vi "MainLogging.vi"() -> ()   [LabVIEW 2020]
uses:
  510ae374-dab3-4fa4-a969-3b7666ba4ceb.vi
  5b4dafd0-0cd6-4d81-9f73-653c943f8121.vi
  <vilib>/Array/Sort 2D Array - Pop Stack.vi
  <vilib>/Array/Sort 2D Array - Push Stack.vi
  510ae374-dab3-4fa4-a969-3b7666ba4ceb.vi/269d4b3b-47f5-49e3-8884-44851e4dd9d5.vi
  510ae374-dab3-4fa4-a969-3b7666ba4ceb.vi/6d99389c-673d-4efb-bf33-19b32bcf4cf8.vi
  5b4dafd0-0cd6-4d81-9f73-653c943f8121.vi/269d4b3b-47f5-49e3-8884-44851e4dd9d5.vi
  5b4dafd0-0cd6-4d81-9f73-653c943f8121.vi/6d99389c-673d-4efb-bf33-19b32bcf4cf8.vi
  Global Variables/Global Enable Logging.vi
panel:
  out "Logging":bool
  out "Display Duration":dbl[](array[numeric])
  out "Square Timestamp":dbl[](array[numeric])
  out "Square Position":dbl[](array[numeric])
  out "Square Size":dbl[](array[numeric])
  out "Avg Pupil Size Right Before NN":dbl[](array[numeric])
  out "Avg Pupil Size Left Before NN":dbl[](array[numeric])
  out "Answer":dbl[](array[numeric])
  out "Label":dbl[](array[numeric])
  out "Classification":dbl[](array[numeric])
  out "Frame Rate":dbl[](array[numeric])
  out "Window Size":dbl[](array[numeric])
  out "Right Pupil Window Avg":dbl[](array[numeric])
  out "Left Pupil Window Avg":dbl[](array[numeric])
  out "Window TimeStamp":dbl[](array[numeric])
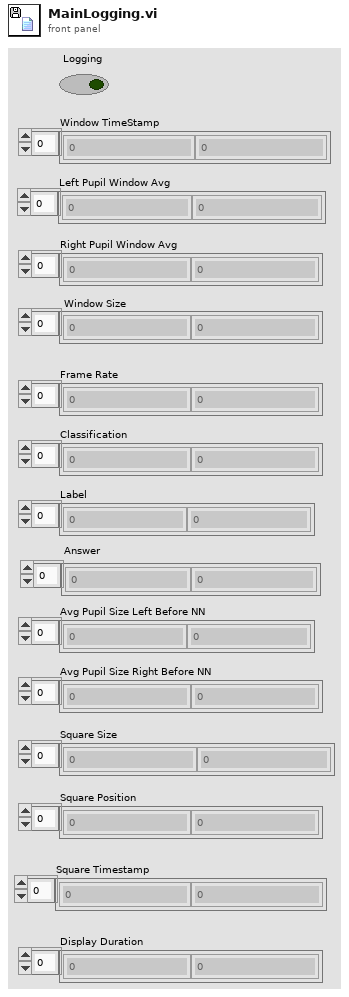
[diagram p1: front panel]
types:
  T1 = enum16{"open", "replace", "create", "open or create", "replace or create", "replace or create with confirmation"}
  T2 = cluster{"[0]":refnum<file>, "[1]":refnum<file>, "[2]":refnum<file>, "[3]":refnum<file>, "[4]":refnum<file>, "[5]":refnum<file>, "[6]":refnum<file>, "[7]":refnum<file>, "[8]":refnum<file>, "[9]":refnum<file>, "[10]":refnum<file>, "[11]":refnum<file>, "[12]":refnum<file>, "[13]":refnum<file>, "[14]":refnum<file>}
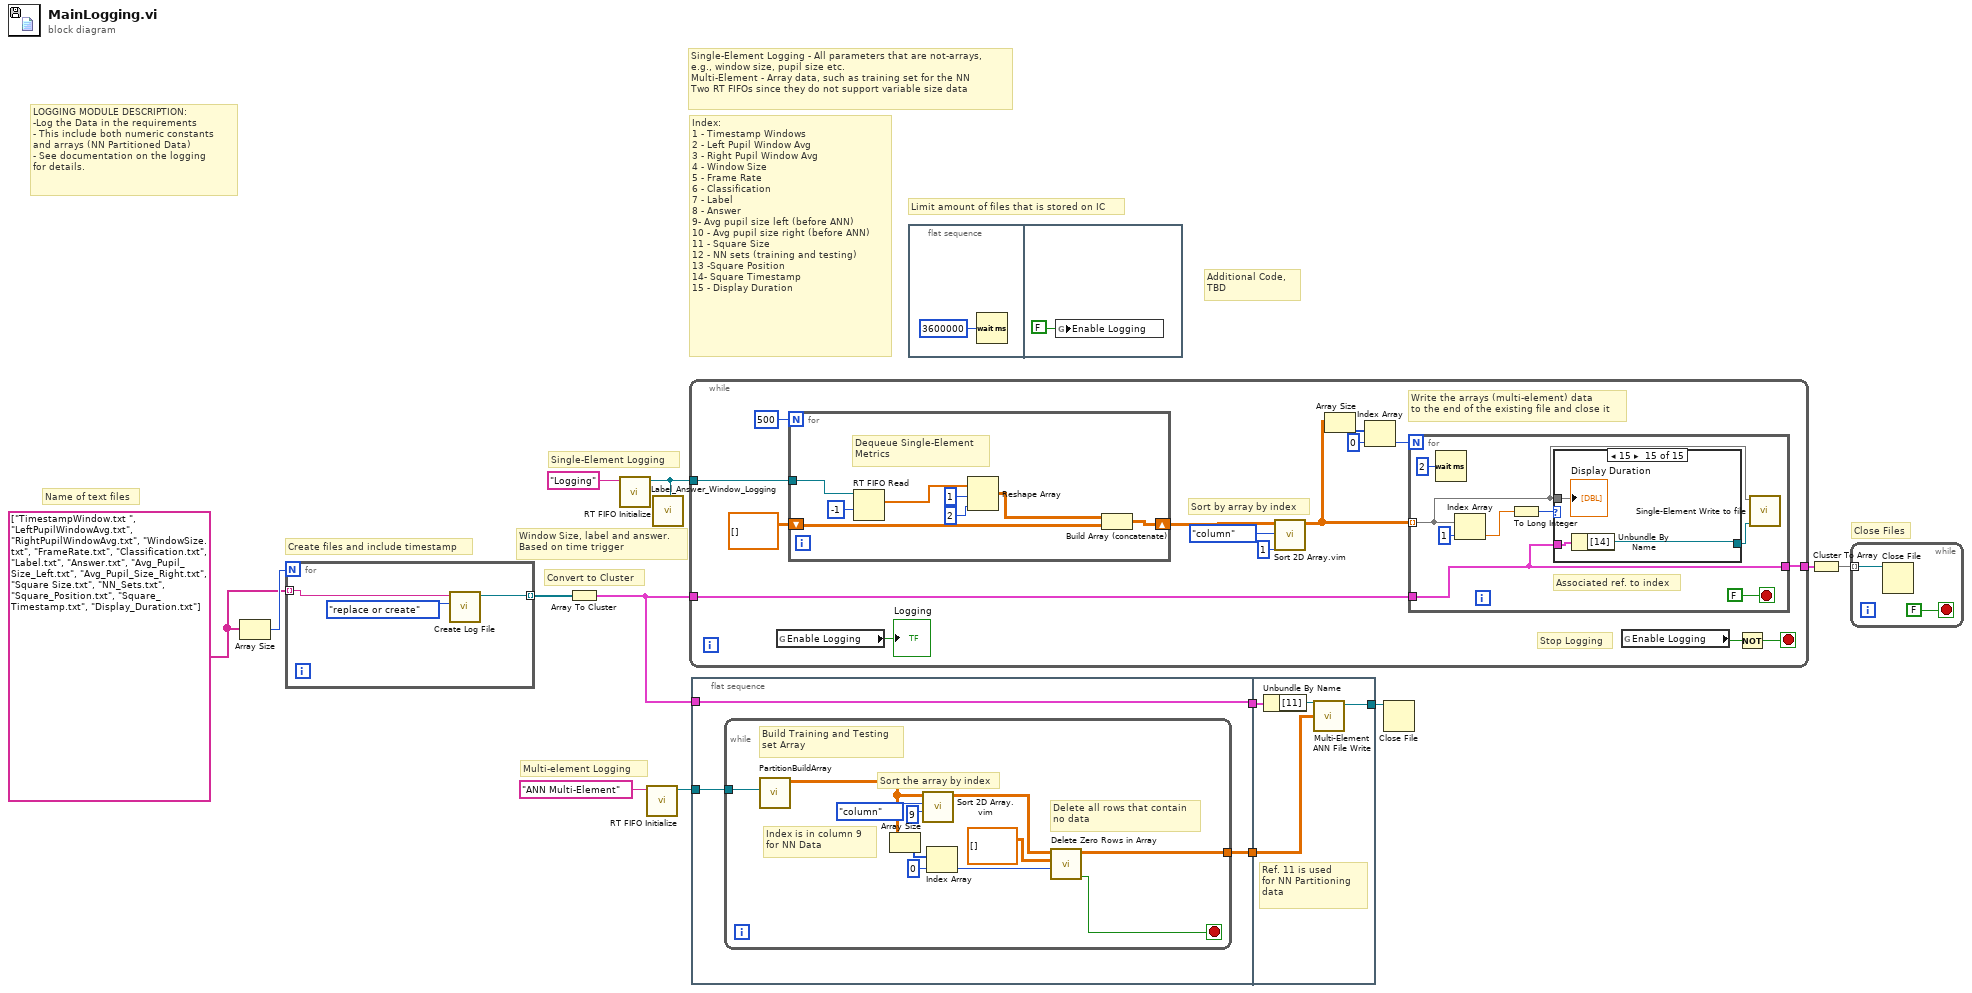
[diagram p0: block diagram]
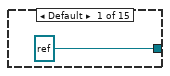
[diagram p2: hidden frame]
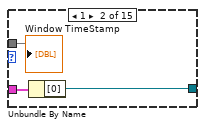
[diagram p3: hidden frame]
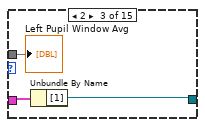
[diagram p4: hidden frame]
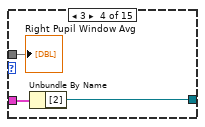
[diagram p5: hidden frame]
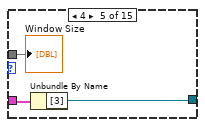
[diagram p6: hidden frame]
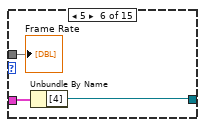
[diagram p7: hidden frame]
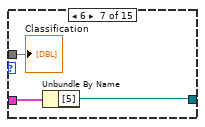
[diagram p8: hidden frame]
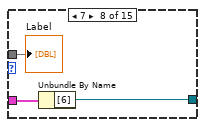
[diagram p9: hidden frame]
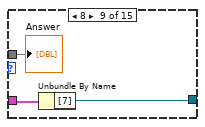
[diagram p10: hidden frame]
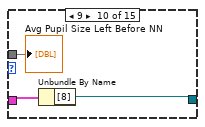
[diagram p11: hidden frame]
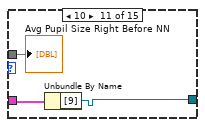
[diagram p12: hidden frame]
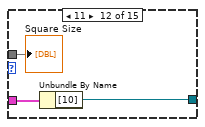
[diagram p13: hidden frame]
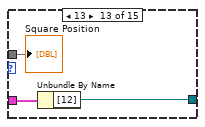
[diagram p14: hidden frame]
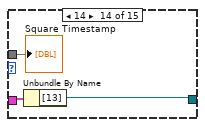
[diagram p15: hidden frame]
diagram:
  w8 = string[] ["TimestampWindow.txt ", "LeftPupilWindowAvg.txt", "RightPupilWindowAvg.txt", "WindowSize.txt", "FrameRate.txt", "Classification.txt", "Label.txt", "Answer.txt", "Avg_Pupil_Size_Left.txt", "Avg_Pupil_Size_Right.txt", "Square Size.txt", "NN_Sets.txt", "Square_Position.txt", "Square_Timestamp.txt", "Display_Duration.txt"]
  # "Close Files"
  # "LOGGING MODULE DESCRIPTION: \n-Log the Data in the requirements \n- This include both numeric constants \nand arrays (NN Partitioned Data) \n- See documentation on the logging \nfor details."
  # "Convert to Cluster"
  # "Additional Code, \nTBD"
  # "Name of text files"
  # "Multi-element Logging"
  # "Create files and include timestamp"
  # "Limit amount of files that is stored on IC"
  # "Window Size, label and answer. \nBased on time trigger"
  # "Single-Element Logging - All parameters that are not-arrays, \ne.g., window size, pupil size etc. \nMulti-Element - Array data, such as training set for the NN \nTwo RT FIFOs since they do not support variable size data"
  # "Single-Element Logging"
  # "Index: \n1 - Timestamp Windows \n2 - Left Pupil Window Avg \n3 - Right Pupil Window Avg\n4 - Window Size\n5 - Frame Rate\n6 - Classification\n7 - Label \n8 - Answer \n9- Avg pupil size left (before ANN) \n10 - Avg pupil size right (before ANN)\n11 - Square Size\n12 - NN sets (training and testing) \n13 -Square Position \n14- Square Timestamp\n15 - Display Duration"
  n1 = Array Size(array=w8) -> (size(s)=w12:i32)
  n2 = for {
    N: w12 -> [_]
    tunnel: [w15] -> w10 mode=indexing
    tunnel: w8 -> [w14] mode=indexing
    n3 = call "Create Log File.vi"("Mode"=T1."replace or create" ("operation (0:open)"), "string"=w14) -> ("Byte Stream File out"=w15:refnum<file>)  [unwired: 8 in, 1 out]
  }
  n4 = Array To Cluster(array=w10) -> (cluster=w4:T2)
  n5 = call "RT FIFO Initialize.vi"("name (unnamed)"="Logging") -> ("rt fifo"=w11:refnum<k33>)  [unwired: 9 in, 1 out]
  n6 = call "RT FIFO Initialize.vi"("name (unnamed)"="ANN Multi-Element") -> ("rt fifo"=w6:refnum<k33>)  [unwired: 9 in, 1 out]
  n7 = call "Label_Answer_Window_Logging.vi"("rt fifo"=w11) -> ()  [unwired: 11 in]
  n8 = while {
    tunnel: w11 -> [w20]
    tunnel: [w22] -> w9
    tunnel: w4 -> [w21]
    stop <- w19 stop-if-true
    # "Stop Logging"
    # "Sort by array by index"
    # "Write the arrays (multi-element) data \nto the end of the existing file and close it"
    n9 = global read "Global Enable Logging.vi" "Enable Logging"() -> (→"Logging":bool)
    n10 = for {
      N: 500 -> [_]
      tunnel: w20 -> [w90]
      shift-right: [w83] -> w28
      shift-left: dbl[][] [] ("sorted 2D array") -> [w88]
      # "Dequeue Single-Element \nMetrics"
      n11 = RT FIFO Read(0:w90, 2:-1 ("timeout in ms (0)")) -> (9:w87:sgl[])  [unwired: 2 in, 4 out]
      n12 = Reshape Array(w87, 1 ("dimension size"), 2 ("dimension size")) -> (w85:sgl[][])
      n13 = Build Array (concatenate)(w85, w88) -> (w83:dbl[][])
    }
    n14 = call "Sort 2D Array.vim"("index"=1, "dimension to index (column)"=enum16{"column", "row"}."column", "2D array"=w28) -> ("sorted 2D array"=w27:dbl[][])  [unwired: 7 in, 1 out]
    n15 = Array Size(array=w27) -> (size(s)=w30:i32[])
    n16 = Index Array(array=w30, index=0) -> (element=w23:i32)
    n17 = for {
      N: w23 -> [_]
      tunnel: w27 -> [w33] mode=indexing
      tunnel: w21 -> [w35]
      tunnel: [w35] -> w22
      stop <- FALSE stop-if-true
      # "Associated ref. to index"
      n18 = Wait (ms)(milliseconds to wait=u32 2) -> ()  [unwired: 1 out]
      n19 = Index Array(array=w33, index=1) -> (element=w36:dbl)
      n20 = To Long Integer(number=w36) -> (32bit integer=w37:i32)
      n21 = case shown="15" w37 {
        tunnel: w35 -> [_ w43 w46 w48 w51 w55 w58 w60 w63 w66 w69 w73 w76 w79 w82]
        tunnel: [refnum<file> refnum ("[9]") w42 w45 w49 w52 w54 w57 w61 w64 w67 w70 w72 w75 w78 w81] -> w32
        tunnel: w33 -> [_ w41 w44 w47 w50 w53 w56 w59 w62 w65 w68 w71 w74 w77 w80]
        frame Default {
        }
        frame 1 {
          n22 = Unbundle By Name(w43) -> ("[0]"=w42:refnum<file>)
          "Window TimeStamp" <- w41
        }
        frame 2 {
          n23 = Unbundle By Name(w46) -> ("[1]"=w45:refnum<file>)
          "Left Pupil Window Avg" <- w44
        }
        frame 3 {
          n24 = Unbundle By Name(w48) -> ("[2]"=w49:refnum<file>)
          "Right Pupil Window Avg" <- w47
        }
        frame 4 {
          n25 = Unbundle By Name(w51) -> ("[3]"=w52:refnum<file>)
          "Window Size" <- w50
        }
        frame 5 {
          n26 = Unbundle By Name(w55) -> ("[4]"=w54:refnum<file>)
          "Frame Rate" <- w53
        }
        frame 6 {
          n27 = Unbundle By Name(w58) -> ("[5]"=w57:refnum<file>)
          "Classification" <- w56
        }
        frame 7 {
          n28 = Unbundle By Name(w60) -> ("[6]"=w61:refnum<file>)
          "Label" <- w59
        }
        frame 8 {
          n29 = Unbundle By Name(w63) -> ("[7]"=w64:refnum<file>)
          "Answer" <- w62
        }
        frame 9 {
          n30 = Unbundle By Name(w66) -> ("[8]"=w67:refnum<file>)
          "Avg Pupil Size Left Before NN" <- w65
        }
        frame 10 {
          n31 = Unbundle By Name(w69) -> ("[9]"=w70:refnum<file>)
          "Avg Pupil Size Right Before NN" <- w68
        }
        frame 11 {
          n32 = Unbundle By Name(w73) -> ("[10]"=w72:refnum<file>)
          "Square Size" <- w71
        }
        frame 13 {
          n33 = Unbundle By Name(w76) -> ("[12]"=w75:refnum<file>)
          "Square Position" <- w74
        }
        frame 14 {
          n34 = Unbundle By Name(w79) -> ("[13]"=w78:refnum<file>)
          "Square Timestamp" <- w77
        }
        frame 15 {
          n35 = Unbundle By Name(w82) -> ("[14]"=w81:refnum<file>)
          "Display Duration" <- w80
        }
      }
      n36 = call "Single-Element Write to file.vi"("refnum"=w32, "sorted 2D array"=w33) -> ()  [unwired: 7 in, 2 out]
    }
    n37 = global read "Global Enable Logging.vi" "Enable Logging"() -> (w18:bool)
    n38 = Not(x=w18) -> (.not. x?=w19:bool)
  }
  n39 = flat-sequence {
    tunnel: w6 -> [w93]
    tunnel: [w92] -> w5
    tunnel: w4 -> [w92]
    tunnel: [w91] -> w2
    tunnel: w5 -> [w108]
    tunnel: [w106] -> w3
    tunnel: w2 -> [w105]
    frame #0 {
      n40 = while {
        tunnel: w93 -> [w104]
        tunnel: [w95] -> w91
        stop <- w94 stop-if-true
        # "Index is in column 9 \nfor NN Data"
        # "Build Training and Testing \nset Array"
        # "Delete all rows that contain \nno data"
        # "Sort the array by index"
        n41 = call "PartitionBuildArray.vi"("rt fifo"=w104) -> ("NN Set Check"=w96:sgl[][])  [unwired: 9 in, 1 out]
        n42 = Array Size(array=w96) -> (size(s)=w99:i32[])
        n43 = call "Sort 2D Array.vim"("index"=9, "dimension to index (column)"=enum16{"column", "row"}."column", "2D array"=w96) -> ("sorted 2D array"=w101:sgl[][])  [unwired: 7 in, 1 out]
        n44 = Index Array(array=w99, index=0) -> (element=w97:i32)
        n45 = call "Delete Zero Rows in Array.vi"("Array Size"=w97, "Initialized Array"=sgl[][] [], "Sorted 2D array"=w101) -> ("Boolean"=w94:bool, "Array out"=w95:sgl[][])  [unwired: 7 in]
      }
    }
    frame #1 {
      # "Ref. 11 is used \nfor NN Partitioning \ndata"
      n46 = Unbundle By Name(w108) -> ("[11]"=w107:refnum<file>)
      n47 = call "Multi-Element ANN File Write.vi"("Array In"=w105, "Training refnum"=w107) -> ("refnum out"=w106:refnum<file>)  [unwired: 8 in, 1 out]
    }
  }
  n48 = flat-sequence {
    frame #0 {
      n49 = Wait (ms)(milliseconds to wait=u32 3600000) -> ()  [unwired: 1 out]
    }
    frame #1 {
      n50 = global write "Global Enable Logging.vi" "Enable Logging"(FALSE ("Stop Logging (automatic)")) -> ()
    }
  }
  n51 = Close File(refnum=w3) -> ()  [unwired: 1 in, 2 out]
  n52 = Cluster To Array(cluster=w9) -> (array=w1:refnum<file>[])
  n53 = while {
    tunnel: w1 -> [w112] mode=indexing
    stop <- FALSE stop-if-true
    n54 = Close File(refnum=w112) -> ()  [unwired: 1 in, 2 out]
  }
